vi "GalilServerCom.vi"(0 "Input":string) -> (1 "Output":string, 2 "error out":errorcluster)   [LabVIEW 2011]
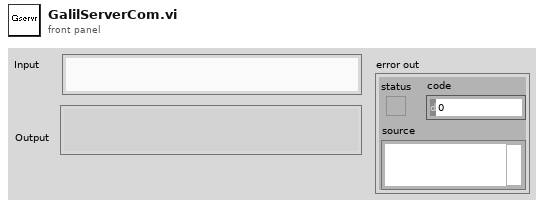
[diagram p1: front panel]
types:
  T1 = enum16{"Standard", "Buffered", "CRLF", "Immediate"}
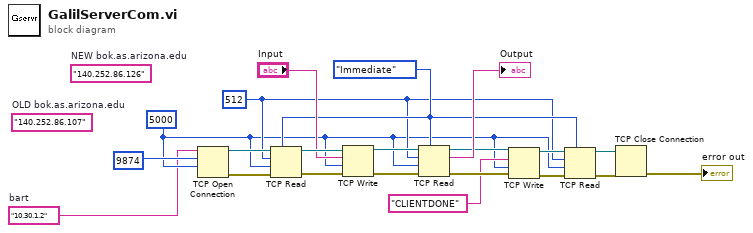
[diagram p0: block diagram]
diagram:
  w1 = "10.30.1.2"  # bart
  (unwired) "140.252.86.107"  # OLD bok.as.arizona.edu
  w6 = T1."Immediate" ("mode (standard)")
  w2 = 5000 ("timeout ms (60000)")
  w5 = 512
  (unwired) "140.252.86.126"  # NEW bok.as.arizona.edu
  n1 = TCP Open Connection(address=w1, remote port or service name=u16 9874 ("remote port"), timeout ms (60000)=w2) -> (connection ID=w17:refnum<k5>, error out=w16:errorcluster)  [unwired: 2 in]
  n2 = TCP Read(connection ID=w17, bytes to read=w5, error in (no error)=w16, 7:w6, 9:w2) -> (connection ID out=w14:refnum<k5>, error out=w15:errorcluster)  [unwired: 1 out]
  n3 = TCP Write(connection ID=w14, data in="Input", error in (no error)=w15, 9:w2) -> (connection ID out=w20:refnum<k5>, error out=w19:errorcluster)  [unwired: 1 out]
  n4 = TCP Read(connection ID=w20, bytes to read=w5, error in (no error)=w19, 7:w6, 9:w2) -> (connection ID out=w13:refnum<k5>, data out=→"Output":string, error out=w12:errorcluster)
  n5 = TCP Write(connection ID=w13, data in="CLIENTDONE", error in (no error)=w12, 9:w2) -> (connection ID out=w11:refnum<k5>, error out=w4:errorcluster)  [unwired: 1 out]
  n6 = TCP Read(connection ID=w11, bytes to read=w5, error in (no error)=w4, 7:w6, 9:w2) -> (connection ID out=w9:refnum<k5>, error out=w10:errorcluster)  [unwired: 1 out]
  n7 = TCP Close Connection(connection ID=w9, error in (no error)=w10) -> (error out=→"error out":errorcluster)  [unwired: 1 in, 1 out]
